vi "Read RP transceiver.vi"(8 "error in (no error)":errorcluster, 11 "Spectrum Recorder too in":refnum<class "Spectrum Recorder too.lvclass">) -> (0 "error out":errorcluster, 2 "RP Transceiver.lvclass":refnum<class "RP Transceiver.lvclass">, 3 "Spectrum Recorder too out":refnum<class "Spectrum Recorder too.lvclass">)   [LabVIEW 2016, in "Spectrum Recorder too.lvclass"]
uses:
  Spectrum Recorder too.lvclass
  C:/github/LabActor/Instrument Actor/Instrument Actor.lvclass
  NHMFL_Core/Libraries/Red Pitaya/RP Core/RP Transceiver/RP Transceiver.lvclass
  Instrument Actor/Instrument Actor.lvclass/Instrument Actor.ctl
  NHMFL_Core/Libraries/Red Pitaya/RP Core/Red Pitaya Transceiver Driver/Red Pitaya Transceiver Driver.lvclass
  NHMFL_Core/Libraries/Red Pitaya/RP Core/Red Pitaya Transceiver Driver/Red Pitaya Transceiver Driver.lvclass/Red Pitaya Transceiver Driver.ctl
  Instrument Actor/Read Instrument driver.vi
  NHMFL_Core/Libraries/Red Pitaya/RP Core/Red Pitaya Transceiver Driver/Read RP Transceiver.vi
  NHMFL_Core/Libraries/Instruments/Instrument Driver/Instrument Driver.lvclass
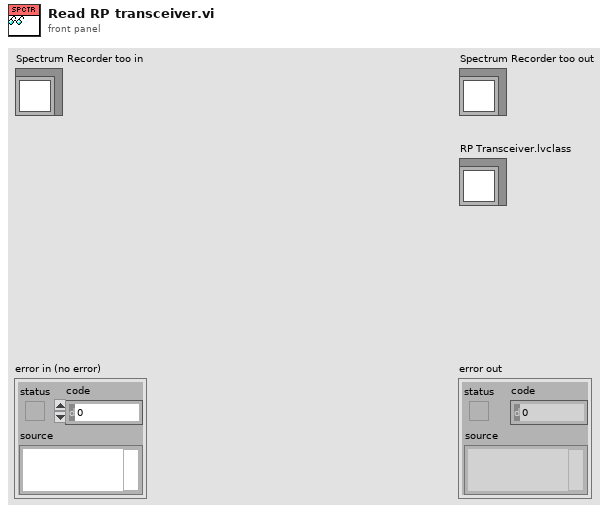
[diagram p1: front panel]
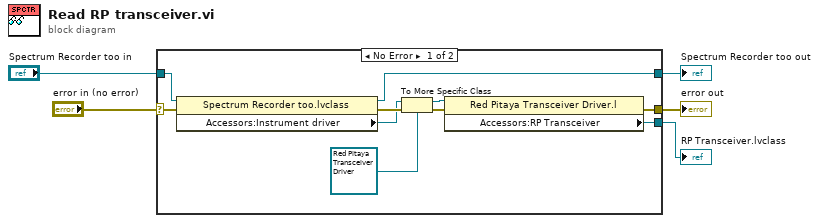
[diagram p0: block diagram]
diagram:
  n1 = case shown="No Error" "error in (no error)" {
    selector: "error in (no error)" -> [w9 w16]
    tunnel: [w8 w16] -> w4
    tunnel: [w6 w17] -> w2
    tunnel: "Spectrum Recorder too in" -> [w7 w17]
    tunnel: [w10 _] -> w1
    frame No Error {
      n2 = property class="Spectrum Recorder too.lvclass"(reference=w7, error in=w9) -> (reference out=w6:refnum<class "Spectrum Recorder too.lvclass">, error out=w14:errorcluster, "Accessors:Instrument driver"=w11:refnum<class "Instrument Driver.lvclass">)
      n3 = To More Specific Class(target class=refnum<class "Red Pitaya Transceiver Driver.lvclass"> refnum ("Red Pitaya Transceiver Driver.lvclass"), reference=w11, error in=w14) -> (specific class reference=w13:refnum<class "Red Pitaya Transceiver Driver.lvclass">, error out=w15:errorcluster)
      n4 = property class="Red Pitaya Transceiver Driver.l"(reference=w13, error in=w15) -> (error out=w8:errorcluster, "Accessors:RP Transceiver"=w10:refnum<class "RP Transceiver.lvclass">)  [unwired: 1 out]
    }
    frame Error {
    }
  }
  "error out" <- w4
  "Spectrum Recorder too out" <- w2
  "RP Transceiver.lvclass" <- w1
